vi "Variant to LV Data.vi"(7 "type":variant, 9 "error in (no error)":errorcluster, 10 "JSON Data in":variant) -> (1 "error out":errorcluster, 2 "Data out":variant)   [LabVIEW 2019, in "Instrument.lvclass"]
doc: "Deprecated in favor of JSON-RPC.lvclass:JSON to LVdata.vi"
uses:
  Instrument.lvclass
  303a33a2-dbc0-401d-b58e-53f0a523a2a2.vi
  <vilib>/Utility/Data Type/NI_Data Type.lvlib
  4d87f6fd-d19c-4d82-9aec-8cbcd500ecd7.vi
  cd7513d2-9d4e-4ca2-b019-c8d72bd8892c.vi
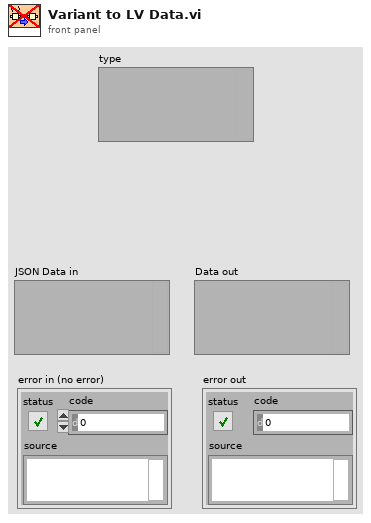
[diagram p1: front panel]
types:
  T1 = typedef "NI_Data Type.lvlib/Data Type.ctl" = enum8{"Invalid Type", "Void", "I8", "I16", "I32", "I64", "U8", "U16", "U32", "U64", "Single Float", "Double Float", "Extended Float", "Single Complex", "Double Complex", "Extended Complex", "Enum U8", "Enum U16", "Enum U32", "Enum U64", "Single Float With Unit", "Double Float With Unit", "Extended Float With Unit", "Single Complex with Unit", "Double Complex with Unit", "Extended Complex with Unit", "Boolean", "String", "Path", "Picture", "Tag", "Array", "Cluster", "Variant", "LV Variant", "Waveform", "Timestamp", "Digital Waveform", "Digital Data", "ExpressData", "Refnum", "External Data", "VI", "Poly VI", "LabVIEW Class Instance", "Fixed Point", "Set Collection", "Map Collection"}
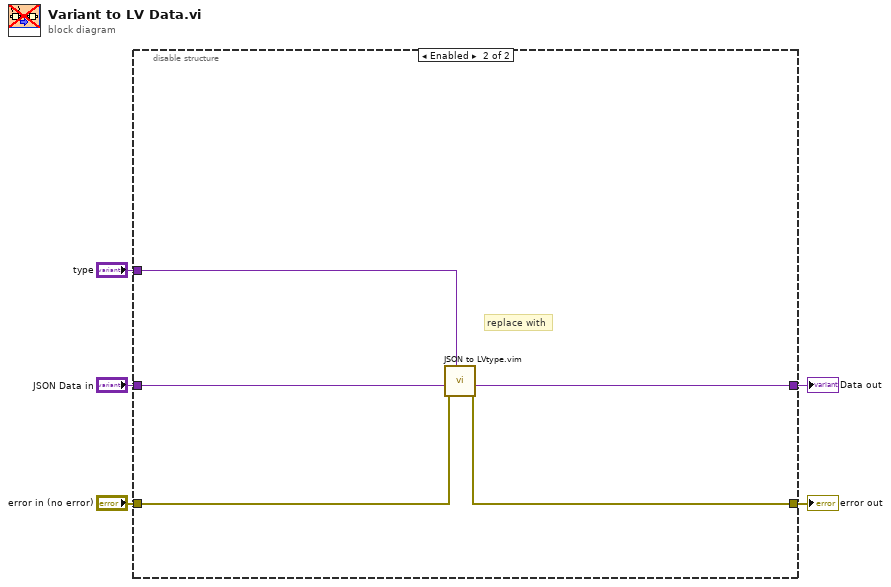
[diagram p0: block diagram]
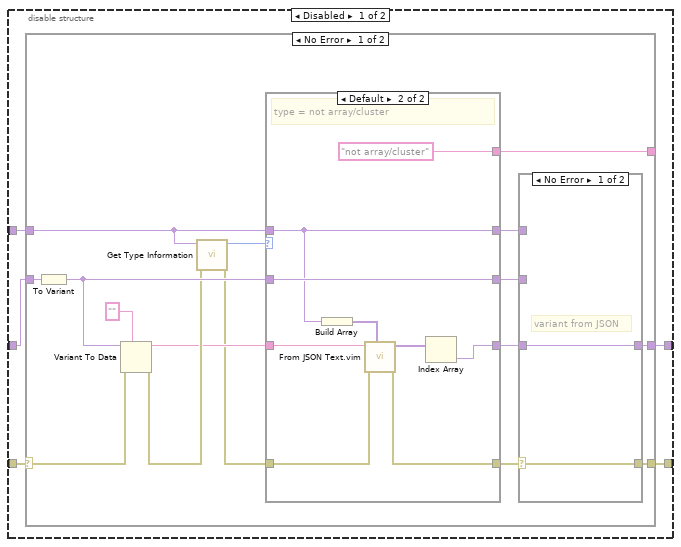
[diagram p2: hidden frame]
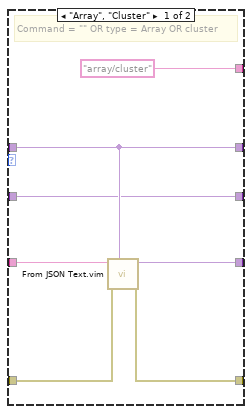
[diagram p3: hidden frame]
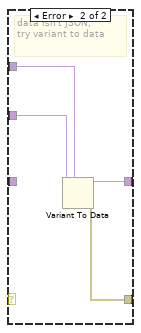
[diagram p4: hidden frame]
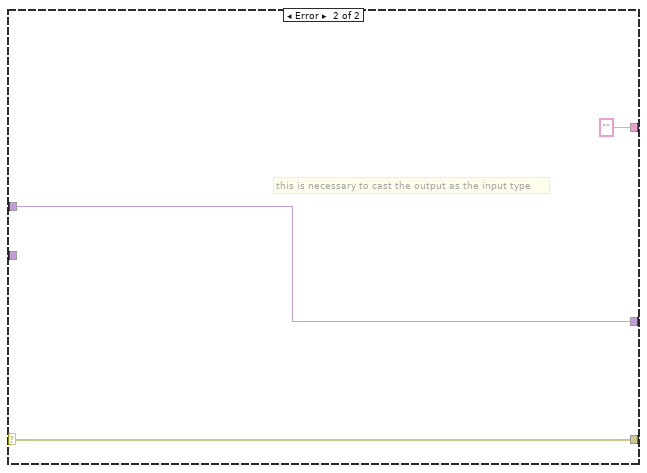
[diagram p5: hidden frame]
diagram:
  n1 = disable-structure shown="Enabled" {
    disable-tunnel: "JSON Data in" -> [w10 w56]
    disable-tunnel: [w9 w55] -> w4
    disable-tunnel: [w8 w54] -> w3
    disable-tunnel: "type" -> [w7 w52]
    disable-tunnel: "error in (no error)" -> [w6 w53]
    frame Disabled {
      n2 = case shown="No Error" w6 {
        selector: w6 -> [w13 w50]
        tunnel: w10 -> [w26 _]
        tunnel: [w25 ""] -> _
        tunnel: [w17 w49] -> w9
        tunnel: [w16 w50] -> w8
        tunnel: w7 -> [w11 w49]
        frame No Error {
          n3 = To Variant(anything=w26) -> (Variant=w24:variant)
          n4 = Variant To Data(error in=w13, type="", Variant=w24) -> (data=w20:string, error out=w21:errorcluster)
          n5 = call <vilib>:"Get Type Information.vi"("error in (no error)"=w21, "variant"=w11) -> ("error out"=w15:errorcluster, "type"=w12:T1)  [unwired: 5 in, 3 out]
          n6 = case shown="Default" w12 {
            tunnel: [w33 w34] -> w18
            tunnel: [w32 w41] -> w23
            tunnel: w20 -> [w31 w40]
            tunnel: w11 -> [w29 w35]
            tunnel: w15 -> [w30 w39]
            tunnel: ["array/cluster" "not array/cluster"] -> w25
            tunnel: [w29 w35] -> w19
            tunnel: [w28 w36] -> w22
            tunnel: w24 -> [w28 w36]
            frame "Array", "Cluster" {
              # "Command = \"\" OR type = Array OR cluster"
              n7 = call "From JSON Text.vim"("Data Type and Default Value"=w29, "error in (no error)"=w30, "JSON"=w31) -> ("error out"=w32:errorcluster, "Data out"=w33:variant)  [unwired: 7 in]
            }
            frame Default {
              # "type = not array/cluster"
              n8 = Build Array(w35) -> (w37:variant[])
              n9 = call "From JSON Text.vim"("Data Type and Default Value"=w37, "error in (no error)"=w39, "JSON"=w40) -> ("error out"=w41:errorcluster, "Data out"=w42:variant[])  [unwired: 7 in]
              n10 = Index Array(array=w42) -> (element=w34:variant)  [unwired: 1 in]
            }
          }
          n11 = case shown="No Error" w23 {
            selector: w23 -> [w43 _]
            tunnel: [w44 w46] -> w17
            tunnel: w18 -> [w44 _]
            tunnel: [w43 w45] -> w16
            tunnel: w22 -> [_ w47]
            tunnel: w19 -> [_ w48]
            frame No Error {
              # "variant from JSON"
            }
            frame Error {
              # "data isn't JSON,\ntry variant to data"
              n12 = Variant To Data(type=w48, Variant=w47) -> (data=w46:variant, error out=w45:errorcluster)  [unwired: 1 in]
            }
          }
        }
        frame Error {
          # "this is necessary to cast the output as the input type"
        }
      }
    }
    frame Enabled {
      # "replace with"
      n13 = call "JSON to LVtype.vim"("type"=w52, "error in (no error)"=w53, "JSON Data in"=w56) -> ("error out"=w54:errorcluster, "Data out"=w55:variant)  [unwired: 7 in]
    }
  }
  "error out" <- w3
  "Data out" <- w4
